vi "Initialize Values Buffer.vi"(10 "channels":T1[](array[typedef]) {"configuration"."string offset" format="%d bytes"}, 11 "values buffer in":u8[](array[numeric])) -> (2 "size":i32, 3 "values buffer out":u8[](array[numeric]))   [LabVIEW 2017, in "DSF Core.lvlib"]
uses:
  DSF Core.lvlib
  Classes/Configuration/Base/Transfer/Channel Configuration.ctl
  Typedefs/Core Channel Configuration.ctl
  Typedefs/DSF Data Type.ctl
  Typedefs/DSF Settings Info.ctl
  Classes/Configuration/Base/Channel/Channel Configuration.lvclass
  Classes/Configuration/Base/Transfer/Transfer Configuration.lvclass
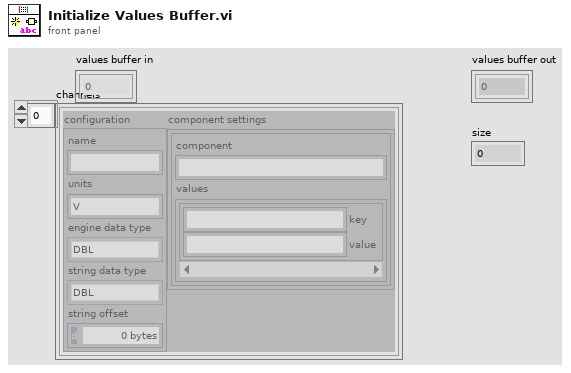
[diagram p1: front panel]
types:
  T1 = typedef "DSF Core.lvlib/Transfer Configuration.lvclass/Channel Configuration.ctl" = cluster{"configuration":T2, "component settings":T4[]}
  T2 = typedef "DSF Core.lvlib/Channel Configuration.lvclass/Core Channel Configuration.ctl" = cluster{"name":string, "units":string, "engine data type":T3, "string data type":T3, "string offset":u64}
  T3 = typedef "DSF Core.lvlib/DSF Data Type.ctl" = enum8{"Bool", "SGL", "DBL", "I8", "I16", "I32", "I64", "U8", "U16", "U32", "U64"}
  T4 = typedef "DSF Core.lvlib/DSF Settings Info.ctl" = cluster{"component":string, "values":cluster{"key":string, "value":string}[]}
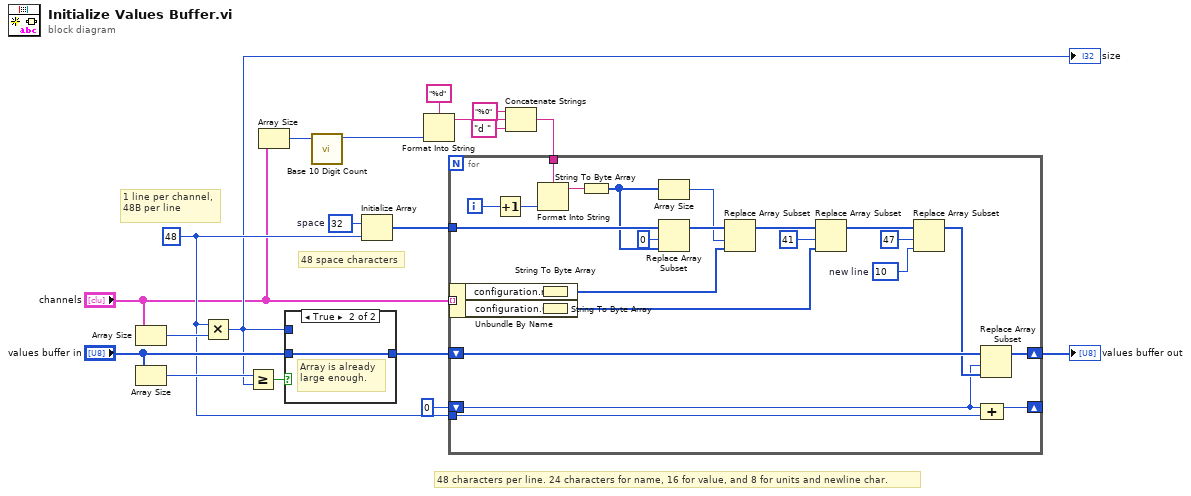
[diagram p0: block diagram]
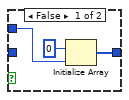
[diagram p2: hidden frame]
diagram:
  w10 = 48 ("x")
  w18 = u8 32  # space
  # "48 characters per line. 24 characters for name, 16 for value, and 8 for units and newline char."
  # "48 space characters"
  # "1 line per channel, 48B per line"
  n1 = Array Size(array="channels") -> (size(s)=w12:i32)
  n2 = Array Size(array="values buffer in") -> (size(s)=w13:i32)
  n3 = Multiply(x=w10, y=w12) -> (x*y=w9:i32)
  "size" <- w9
  n4 = Greater Or Equal?(x=w13, y=w9) -> (x >= y?=w15:bool)
  n5 = Array Size(array="channels") -> (size(s)=w7:i32)
  n6 = case shown="True" w15 {
    tunnel: w9 -> [w20 _]
    tunnel: "values buffer in" -> [_ w23]
    tunnel: [w21 w23] -> w14
    frame False {
      n7 = Initialize Array(u8 0 ("element"), w20) -> (w21:u8[])
    }
    frame True {
      # "Array is already large enough."
    }
  }
  n8 = call "Base 10 Digit Count.vi"("number"=w7) -> ("digit count"=w2:i32)  [unwired: 10 in]
  n9 = Initialize Array(w18, w10) -> (w17:u8[])
  n10 = Format Into String(format string="%d", w2) -> (resulting string=w5:string)  [unwired: 2 in, 1 out]
  n11 = Concatenate Strings("%0" ("string"), w5, "d " ("string")) -> (w1:string)
  n12 = for {
    tunnel: "channels" -> [w48] mode=indexing
    shift-right: [w38] -> w19
    shift-left: w14 -> [w44]
    tunnel: w17 -> [w29]
    shift-right: [w37] -> _
    shift-left: 0 ("x << y") -> [w33]
    tunnel: w10 -> [w36]
    tunnel: w1 -> [w32]
    i -> [w31]
    w39 = u8 10  # new line
    n13 = Unbundle By Name(w48) -> ("configuration.name"=w47:string, "configuration.units"=w45:string)
    n14 = Increment(x=w31) -> (x+1=w24:i32)
    n15 = Format Into String(format string=w32, w24) -> (resulting string=w30:string)  [unwired: 2 in, 1 out]
    n16 = String To Byte Array(string=w47) -> (unsigned byte array=w46:u8[])
    n17 = String To Byte Array(string=w45) -> (unsigned byte array=w34:u8[])
    n18 = String To Byte Array(string=w30) -> (unsigned byte array=w27:u8[])
    n19 = Array Size(array=w27) -> (size(s)=w25:i32)
    n20 = Replace Array Subset(array=w29, new element=w27, index=0) -> (w28:u8[])
    n21 = Replace Array Subset(array=w28, new element=w46, index=w25) -> (w41:u8[])
    n22 = Replace Array Subset(array=w41, new element=w34, index=41) -> (w43:u8[])
    n23 = Replace Array Subset(array=w43, new element=w39, index=47) -> (w35:u8[])
    n24 = Replace Array Subset(array=w44, new element=w35, index=w33) -> (w38:u8[])
    n25 = Compound Arithmetic op=ADD(w33, w36) -> (w37:i32)
  }
  "values buffer out" <- w19
